vi "Plot_RoofShape_Sub.vi"(0 "Selector array In":i32[](array[numeric]), 1 "Mode":T1(ring), 3 "precision":string, 5 "Selector List In":string[](array[string]), 9 "Search String":string, 11 "History (min)":dbl format="%.1f", 14 "End Time":dbl) -> (2 "Position Numbers":dbl[](array[numeric]), 4 "Selector array Out":i32[](array[numeric]), 6 "Selector List Out":string[](array[string]), 10 "Plot":cluster{dbl[], "Output array":dbl[]}(graph), 12 "Selector Changed?":bool, 13 "Position Values":dbl[](array[numeric]), 15 "Plot Legend":string[](array[string]))   [LabVIEW 2020]
uses:
  ADAM Controls/Search_mode.ctl
panel:
  out "Array":dbl[](array[numeric])
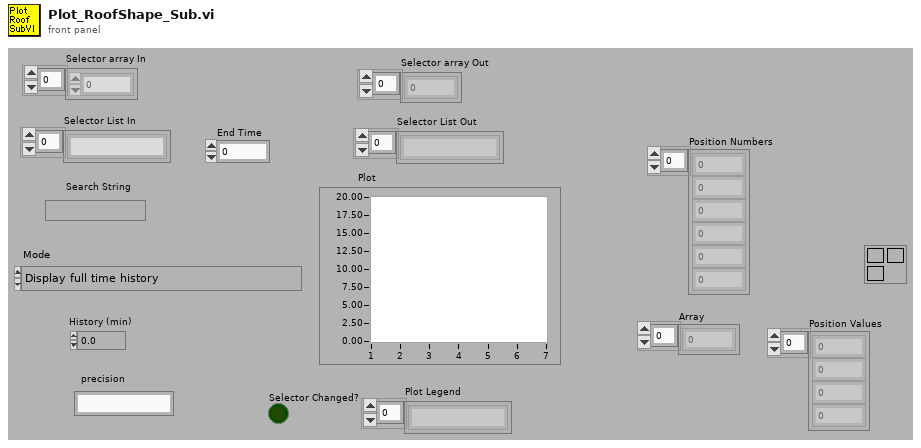
[diagram p1: front panel]
types:
  T1 = enum16{"Display full time history", "Display data over specified period:"}
  T2 = typedef "Search_mode.ctl" = enum16{"Between times", "All Times"}
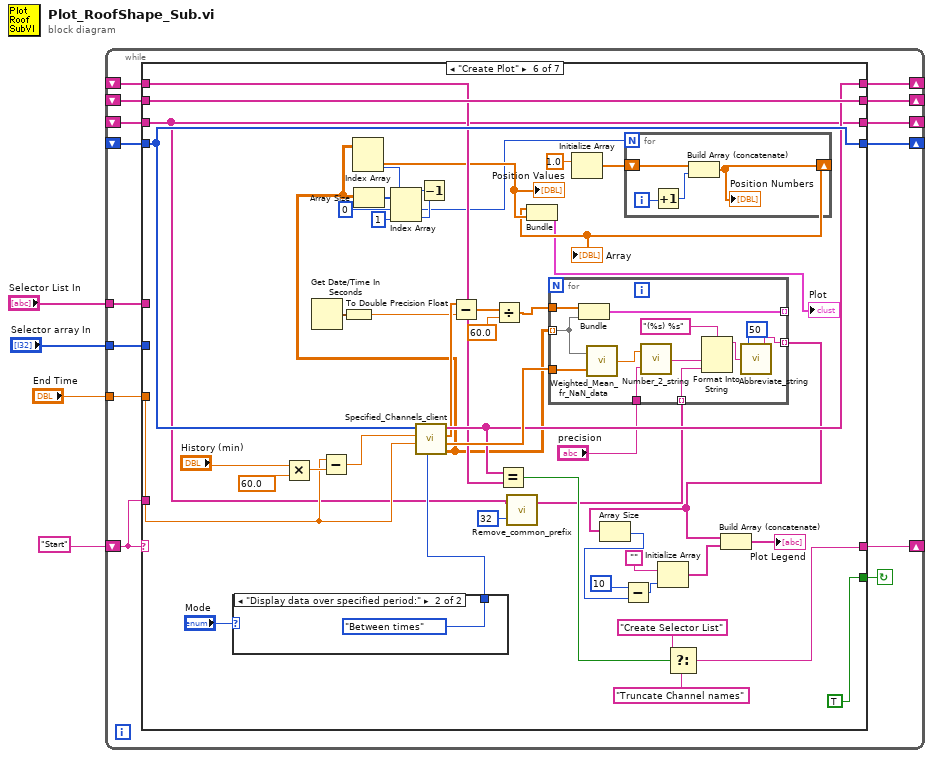
[diagram p0: block diagram]
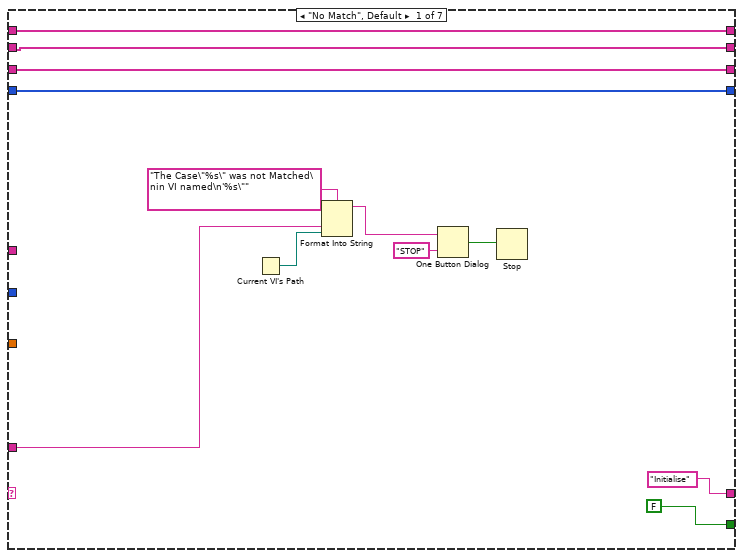
[diagram p2: hidden frame]
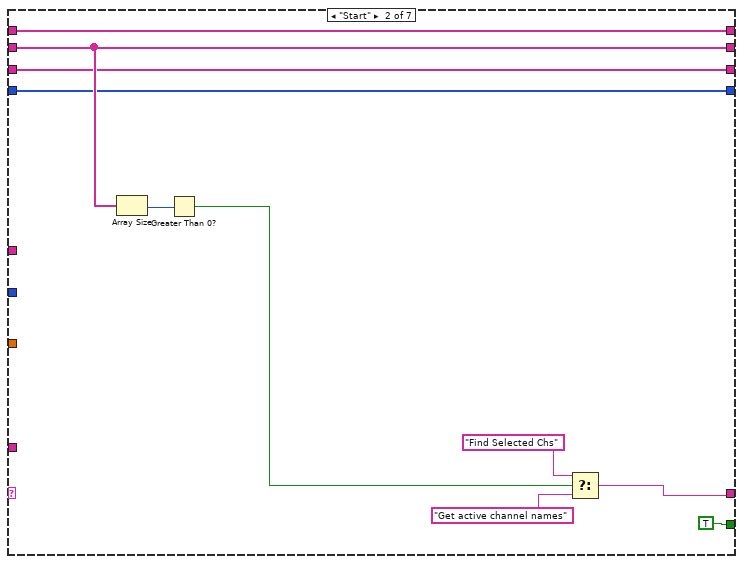
[diagram p3: hidden frame]
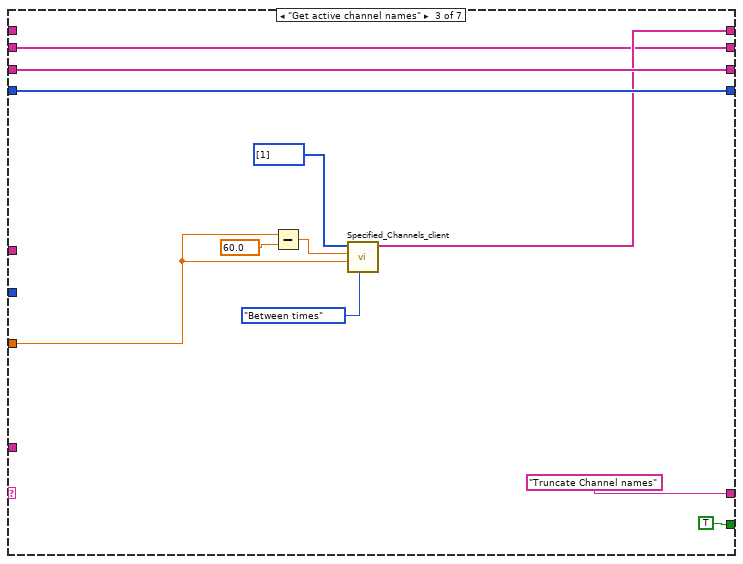
[diagram p4: hidden frame]
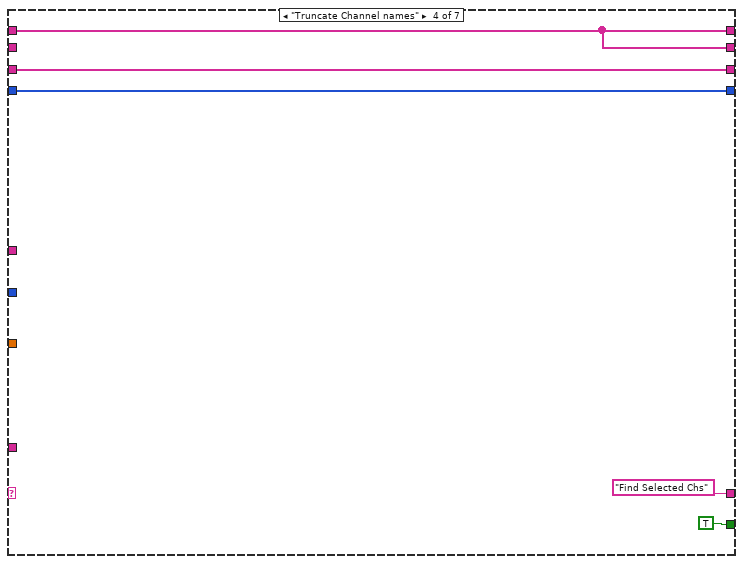
[diagram p5: hidden frame]
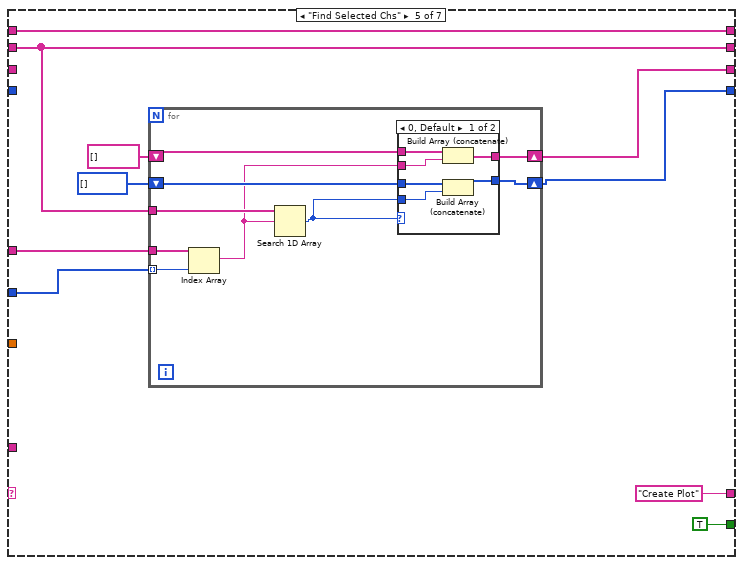
[diagram p6: hidden frame]
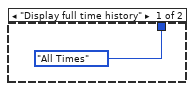
[diagram p8: hidden frame]
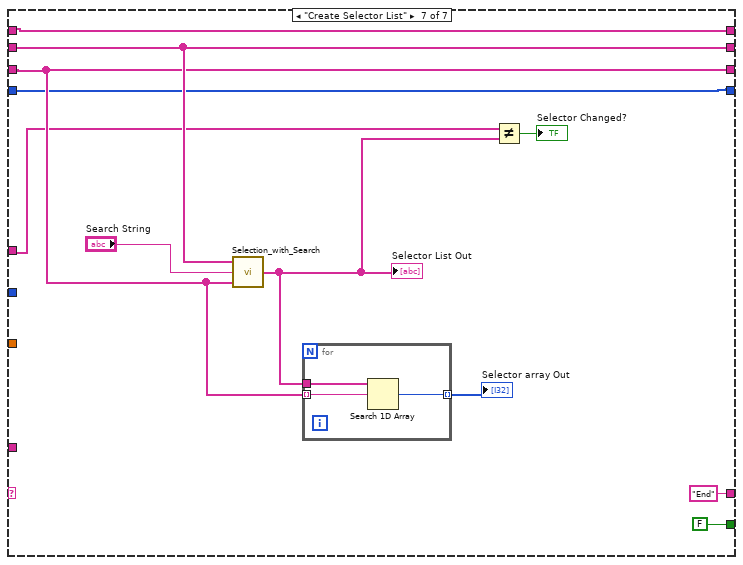
[diagram p9: hidden frame]
diagram:
  n1 = while {
    shift-left: "Start" -> [w16]
    shift-right: [w17] -> _
    shift-right: [w13] -> _
    shift-left: _ -> [w15]
    tunnel: "End Time" -> [w14]
    tunnel: "Selector List In" -> [w12]
    tunnel: "Selector array In" -> [w11]
    shift-right: [w10] -> _
    shift-left: _ -> [w7]
    shift-right: [w9] -> _
    shift-left: _ -> [w8]
    shift-right: [w6] -> _
    shift-left: _ -> [w5]
    stop <- w18 continue-if-true
    n2 = case shown="\"Create Plot\"" w16 {
      tunnel: [FALSE TRUE TRUE TRUE TRUE TRUE FALSE] -> w18
      tunnel: ["Initialise" w35 "Truncate Channel names" "Find Selected Chs" "Create Plot" w114 "End"] -> w17
      tunnel: w16 -> [w25 _ _ _ _ _ _]
      tunnel: w15 -> [w22 w34 w41 _ w62 w120 w157]
      tunnel: w14 -> [_ _ w49 _ _ w111 _]
      tunnel: [w22 w34 w41 w52 w62 w120 w157] -> w13
      tunnel: w12 -> [_ _ _ _ w65 _ w149]
      tunnel: w11 -> [_ _ _ _ w64 _ _]
      tunnel: [w21 w33 w44 w54 w61 w98 w155] -> w10
      tunnel: [w20 w32 w43 w53 w60 w121 w154] -> w9
      tunnel: w8 -> [w20 w32 w43 w53 _ w121 w154]
      tunnel: w7 -> [w21 w33 w44 w54 _ w98 w155]
      tunnel: [w19 w31 w42 w52 w57 w119 w151] -> w6
      tunnel: w5 -> [w19 w31 _ w52 w57 w118 w151]
      frame "No Match", Default {
        n3 = Current VI's Path() -> (path=w24:path)
        n4 = Format Into String(format string="The Case\"%s\" was not Matched\nin VI named\n'%s\"" ("Format String"), w25, w24) -> (resulting string=w28:string)  [unwired: 2 in, 1 out]
        n5 = One Button Dialog(message=w28, button name ("OK")="STOP") -> (true=w26:bool)
        n6 = Stop(stop? (T)=w26) -> ()
      }
      frame "Start" {
        n7 = Array Size(array=w34) -> (size(s)=w39:i32)
        n8 = Greater Than 0?(x=w39) -> (x > 0?=w38:bool)
        n9 = Select(t="Find Selected Chs", s=w38, f="Get active channel names") -> (s? t:f=w35:string)
      }
      frame "Get active channel names" {
        n10 = Subtract(x=w49, y=60.0) -> (x-y=w47:dbl)
        n11 = call "Specified_Channels_client.vi"("Mode"=Search_mode."Between times", "End time"=w49, "Start time"=w47, "ADAM Index array"=i32[] [1]) -> ("All Active Ch Names"=w42:string[])  [unwired: 1 in, 6 out]
      }
      frame "Truncate Channel names" {
      }
      frame "Find Selected Chs" {
        n12 = for {
          tunnel: w62 -> [w75]
          shift-right: [w73] -> w60
          shift-left: i32[] [] -> [w74]
          shift-right: [w68] -> w61
          shift-left: string[] [] -> [w69]
          tunnel: w65 -> [w71]
          tunnel: w64 -> [w70] mode=indexing
          n13 = Index Array(array=w71, index=w70) -> (element=w67:string)
          n14 = Search 1D Array(1D array=w75, element=w67) -> (index of element=w72:i32)  [unwired: 1 out]
          n15 = case shown="0, Default" w72 {
            tunnel: w74 -> [w81 w83]
            tunnel: [w80 w83] -> w73
            tunnel: w72 -> [w79 _]
            tunnel: w69 -> [w78 w82]
            tunnel: [w77 w82] -> w68
            tunnel: w67 -> [w76 _]
            frame 0, Default {
              n16 = Build Array (concatenate)(w78, w76) -> (w77:string[])
              n17 = Build Array (concatenate)(w81, w79) -> (w80:i32[])
            }
            frame -1 {
            }
          }
        }
      }
      frame "Create Plot" {
        n18 = case shown="\"Display data over specified period:\"" "Mode" {
          tunnel: [Search_mode."All Times" ("Mode") Search_mode."Between times" ("Mode")] -> w122
          frame "Display full time history" {
          }
          frame "Display data over specified period:" {
          }
        }
        n19 = Multiply(x="History (min)", y=60.0) -> (x*y=w127:dbl)
        n20 = Get Date/Time In Seconds() -> (seconds since 1Jan1904=w100:timestamp)
        n21 = Subtract(x=w111, y=w127) -> (x-y=w124:dbl)
        n22 = To Double Precision Float(number=w100) -> (double precision float=w99:dbl)
        n23 = call "Specified_Channels_client.vi"("Mode"=w122, "End time"=w111, "Start time"=w124, "ADAM Index array"=w121) -> ("Output array"=w94:dbl[][], "Averaging Period"=w123:dbl[], "Centre Times"=w110:dbl[], "All Active Ch Names"=w119:string[])  [unwired: 1 in, 3 out]
        n24 = Array Size(array=w94) -> (size(s)=w95:i32[])
        n25 = Index Array(array=w95, index #1=0 ("index"), index #2=1 ("index")) -> (element #1=w87:i32, element #2=w89:i32)
        n26 = Decrement(x=w89) -> (x-1=w84:i32)
        n27 = Index Array(array=w94, index (col)=w84) -> (element=w93:dbl[])  [unwired: 1 in]
        "Position Values" <- w93
        n28 = Subtract(x=w110, y=w99) -> (x-y=w113:dbl[])
        n29 = Divide(x=w113, y=60.0) -> (x/y=w109:dbl[])
        n30 = Equal?(x=w119, y=w118) -> (x = y?=w117:bool)
        n31 = call "Remove_common_prefix.vi"("Max String Length"=32, "Array in"=w98) -> ("Array out"=w97:string[])  [unwired: 1 in]
        n32 = for {
          tunnel: w94 -> [w144] mode=indexing
          tunnel: [w145] -> _ mode=indexing
          tunnel: w109 -> [w143]
          tunnel: w123 -> [w142]
          tunnel: w97 -> [w141] mode=indexing
          tunnel: [w137] -> w105 mode=indexing
          tunnel: "precision" -> [w134]
          n33 = Bundle(w143, "Output array"=w144) -> (w145:cluster{dbl[], "Output array":dbl[]})  [unwired: 1 out]
          n34 = call "Weighted_Mean_fr_NaN_data.vi"("Weighting"=w142, "Data"=w144) -> ("Mean value"=w136:dbl)
          n35 = call "Number_2_string.vi"("precision"=w134, "number"=w136) -> ("String"=w135:string)
          n36 = Format Into String(format string="(%s) %s", w135, w141) -> (resulting string=w138:string)  [unwired: 2 in, 1 out]
          n37 = call "Abbreviate_string.vi"("Input String"=w138, "Max String Length"=50) -> ("Output String"=w137:string)  [unwired: 1 in, 2 out]
        }
        n38 = Initialize Array(1.0 ("element")) -> (w91:dbl[])  [unwired: 1 in]
        n39 = Array Size(array=w105) -> (size(s)=w103:i32)
        n40 = Subtract(x=10 ("dimension size"), y=w103) -> (x-y=w102:i32)
        n41 = for {
          N: w87 -> [_]
          shift-right: [w131] -> w86
          shift-left: w91 -> [w132]
          i -> [w133]
          n42 = Increment(x=w133) -> (x+1=w130:i32)
          n43 = Build Array (concatenate)(w132, w130) -> (w131:dbl[])
          "Position Numbers" <- w131
        }
        "Array" <- w86
        n44 = Bundle(w86, "Output array"=w93) -> (→"Plot":cluster{dbl[], "Output array":dbl[]})  [unwired: 1 out]
        n45 = Initialize Array("", w102) -> (w106:string[])
        n46 = Select(t="Create Selector List", s=w117, f="Truncate Channel names") -> (s? t:f=w114:string)
        n47 = Build Array (concatenate)(w105, w106) -> (→"Plot Legend":string[])
      }
      frame "Create Selector List" {
        n48 = call "Selection_with_Search.vi"("Selected Channel Names"=w155, "Search String"="Search String", "All Channel Names"=w157) -> ("Item Names"=w150:string[])
        "Selector List Out" <- w150
        n49 = for {
          tunnel: w150 -> [w161]
          tunnel: w155 -> [w160] mode=indexing
          tunnel: [w159] -> w156 mode=indexing
          n50 = Search 1D Array(1D array=w161, element=w160) -> (index of element=w159:i32)  [unwired: 1 out]
        }
        "Selector array Out" <- w156
        n51 = Not Equal?(x=w149, y=w150) -> (x != y?=→"Selector Changed?":bool)
      }
    }
  }
